vi "150pt Mov Avg.vi"(10 "Value in":dbl) -> (2 "Value out":dbl)   [LabVIEW 2014]
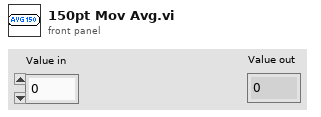
[diagram p1: front panel]
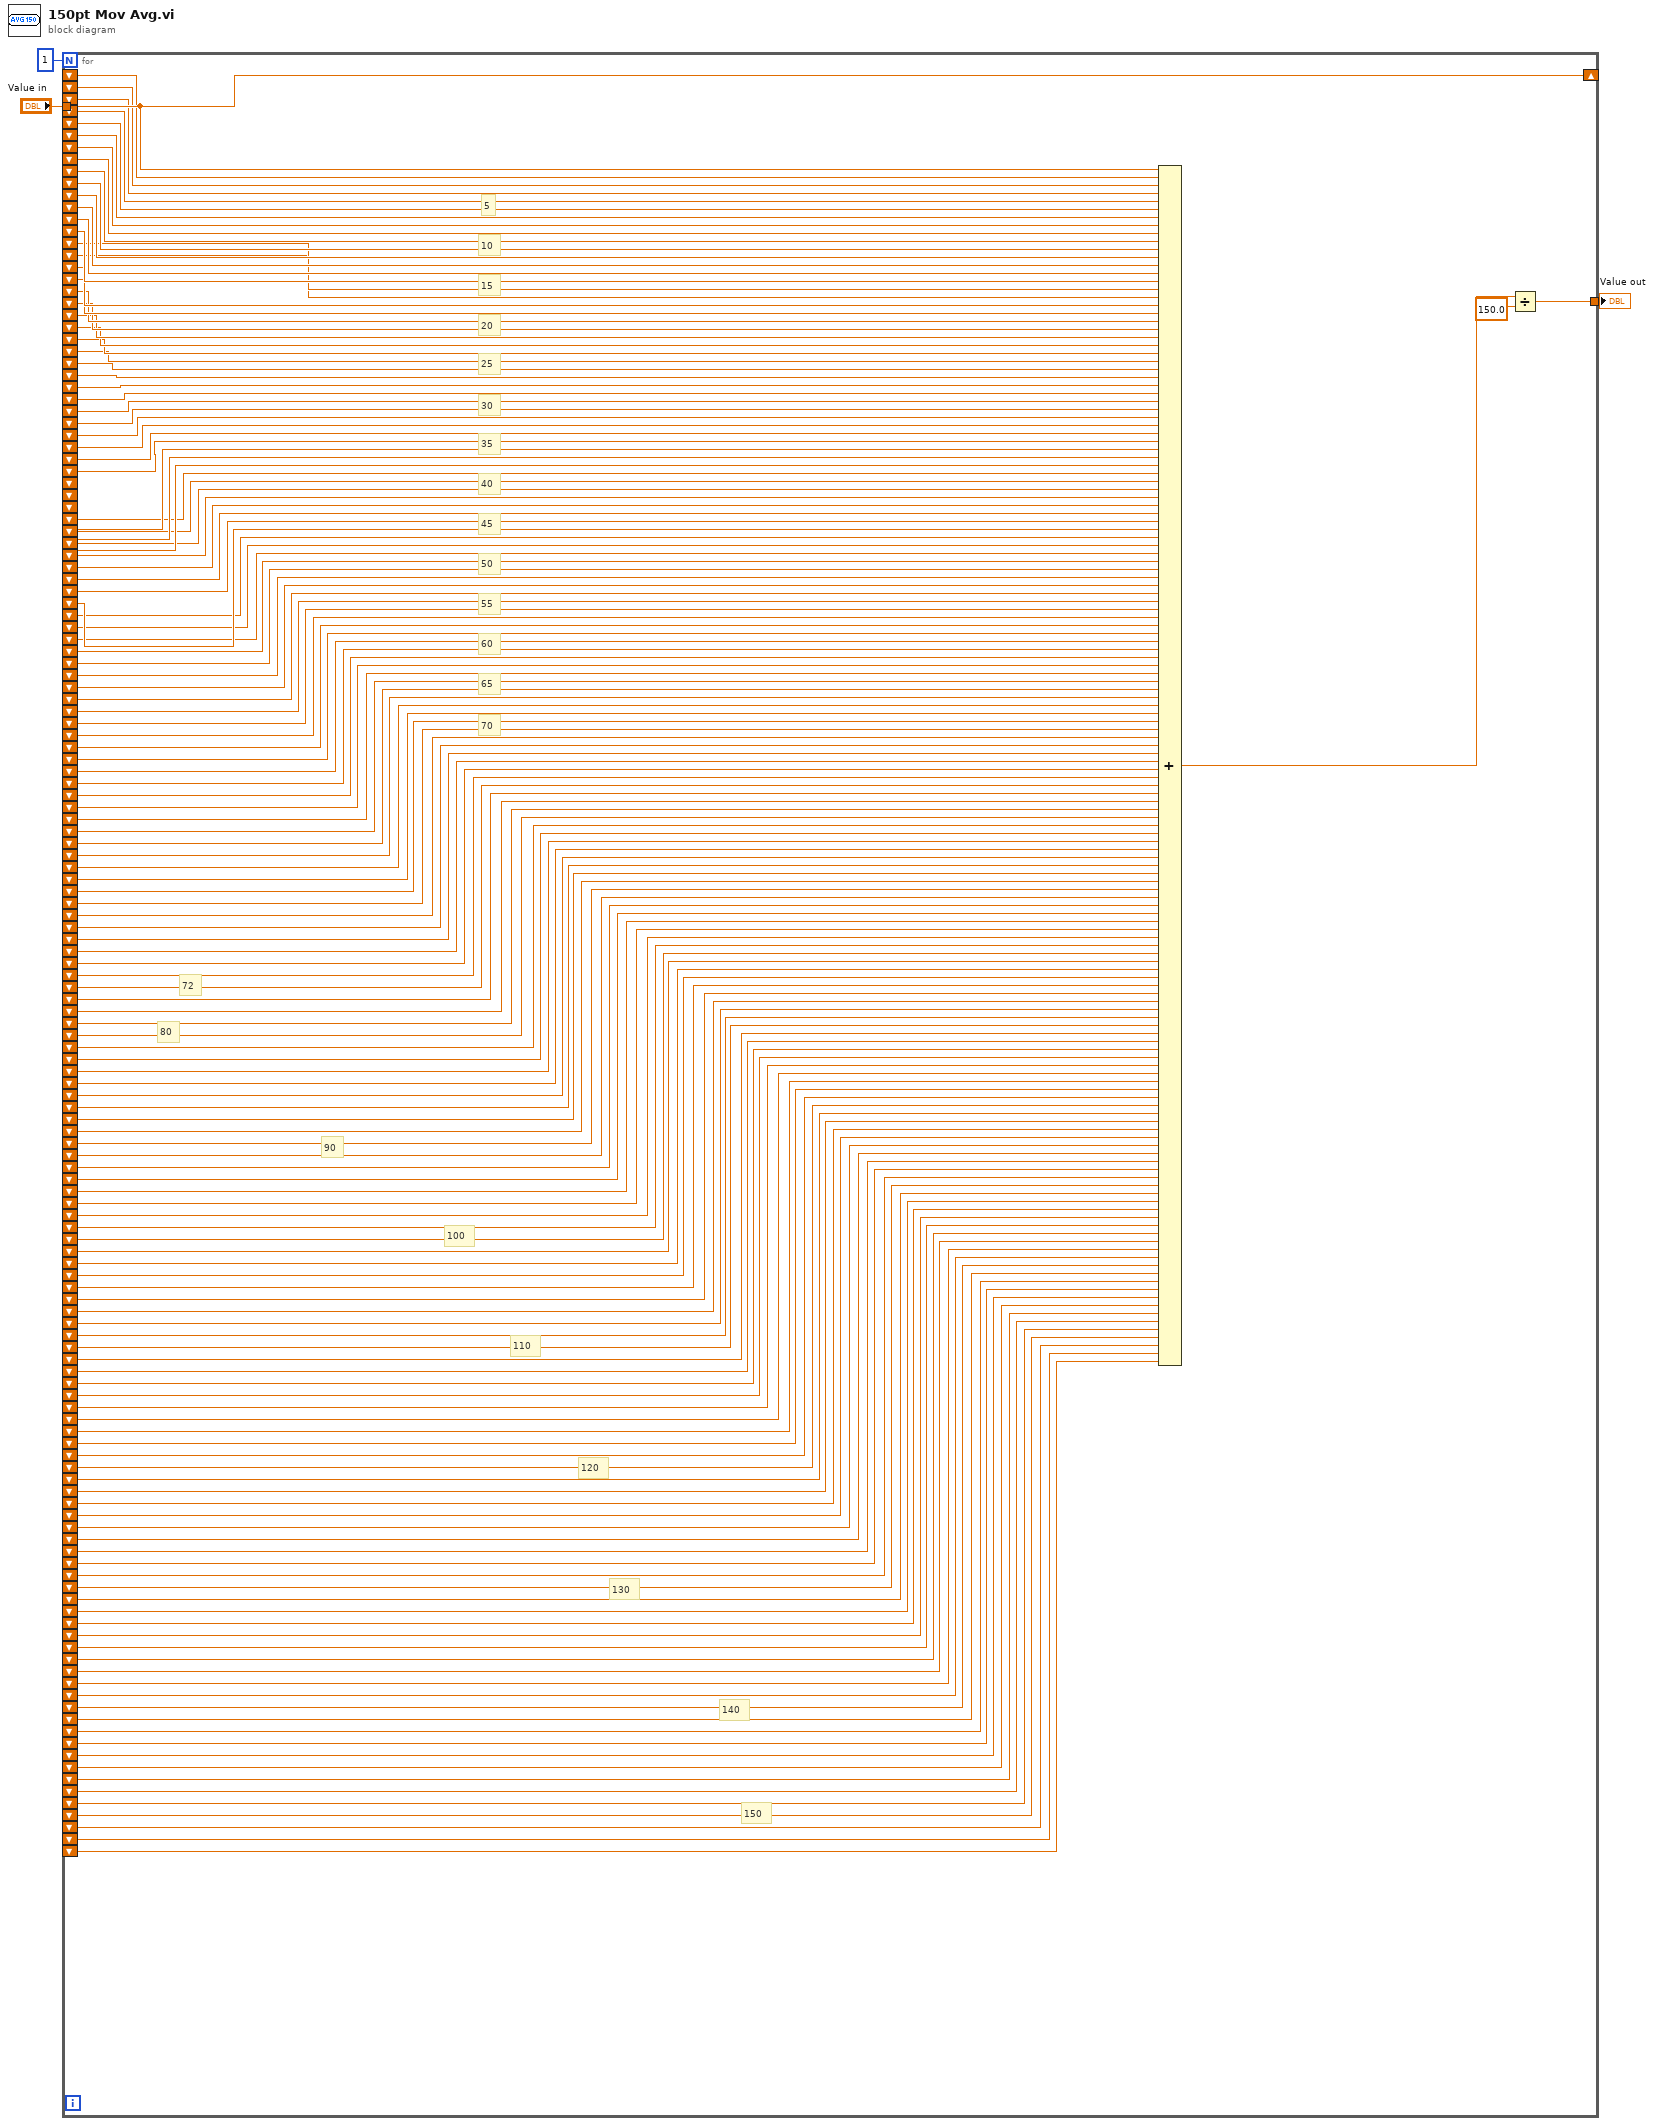
[diagram p0: block diagram]
diagram:
  n1 = for {
    N: 1 -> [_]
    tunnel: "Value in" -> [w156]
    shift-right: [w156] -> _
    shift-left: _ -> [w155]
    shift-left: _ -> [w154]
    shift-left: _ -> [w153]
    shift-left: _ -> [w152]
    tunnel: [w149] -> w1
    shift-left: _ -> [w148]
    shift-left: _ -> [w147]
    shift-left: _ -> [w146]
    shift-left: _ -> [w145]
    shift-left: _ -> [w144]
    shift-left: _ -> [w143]
    shift-left: _ -> [w142]
    shift-left: _ -> [w141]
    shift-left: _ -> [w140]
    shift-left: _ -> [w139]
    shift-left: _ -> [w138]
    shift-left: _ -> [w137]
    shift-left: _ -> [w136]
    shift-left: _ -> [w135]
    shift-left: _ -> [w134]
    shift-left: _ -> [w133]
    shift-left: _ -> [w132]
    shift-left: _ -> [w131]
    shift-left: _ -> [w130]
    shift-left: _ -> [w129]
    shift-left: _ -> [w128]
    shift-left: _ -> [w127]
    shift-left: _ -> [w126]
    shift-left: _ -> [w125]
    shift-left: _ -> [w124]
    shift-left: _ -> [w123]
    shift-left: _ -> [w122]
    shift-left: _ -> [w121]
    shift-left: _ -> [w120]
    shift-left: _ -> [w119]
    shift-left: _ -> [w118]
    shift-left: _ -> [w117]
    shift-left: _ -> [w116]
    shift-left: _ -> [w115]
    shift-left: _ -> [w113]
    shift-left: _ -> [w114]
    shift-left: _ -> [w112]
    shift-left: _ -> [w111]
    shift-left: _ -> [w110]
    shift-left: _ -> [w109]
    shift-left: _ -> [w108]
    shift-left: _ -> [w107]
    shift-left: _ -> [w106]
    shift-left: _ -> [w105]
    shift-left: _ -> [w104]
    shift-left: _ -> [w103]
    shift-left: _ -> [w102]
    shift-left: _ -> [w101]
    shift-left: _ -> [w100]
    shift-left: _ -> [w99]
    shift-left: _ -> [w98]
    shift-left: _ -> [w97]
    shift-left: _ -> [w96]
    shift-left: _ -> [w95]
    shift-left: _ -> [w94]
    shift-left: _ -> [w93]
    shift-left: _ -> [w92]
    shift-left: _ -> [w91]
    shift-left: _ -> [w90]
    shift-left: _ -> [w89]
    shift-left: _ -> [w88]
    shift-left: _ -> [w87]
    shift-left: _ -> [w86]
    shift-left: _ -> [w85]
    shift-left: _ -> [w84]
    shift-left: _ -> [w83]
    shift-left: _ -> [w82]
    shift-left: _ -> [w81]
    shift-left: _ -> [w80]
    shift-left: _ -> [w79]
    shift-left: _ -> [w78]
    shift-left: _ -> [w77]
    shift-left: _ -> [w76]
    shift-left: _ -> [w75]
    shift-left: _ -> [w74]
    shift-left: _ -> [w73]
    shift-left: _ -> [w72]
    shift-left: _ -> [w71]
    shift-left: _ -> [w70]
    shift-left: _ -> [w69]
    shift-left: _ -> [w68]
    shift-left: _ -> [w67]
    shift-left: _ -> [w66]
    shift-left: _ -> [w65]
    shift-left: _ -> [w64]
    shift-left: _ -> [w63]
    shift-left: _ -> [w62]
    shift-left: _ -> [w61]
    shift-left: _ -> [w60]
    shift-left: _ -> [w59]
    shift-left: _ -> [w58]
    shift-left: _ -> [w57]
    shift-left: _ -> [w56]
    shift-left: _ -> [w55]
    shift-left: _ -> [w54]
    shift-left: _ -> [w53]
    shift-left: _ -> [w52]
    shift-left: _ -> [w51]
    shift-left: _ -> [w50]
    shift-left: _ -> [w49]
    shift-left: _ -> [w48]
    shift-left: _ -> [w47]
    shift-left: _ -> [w46]
    shift-left: _ -> [w45]
    shift-left: _ -> [w44]
    shift-left: _ -> [w43]
    shift-left: _ -> [w42]
    shift-left: _ -> [w41]
    shift-left: _ -> [w40]
    shift-left: _ -> [w39]
    shift-left: _ -> [w38]
    shift-left: _ -> [w37]
    shift-left: _ -> [w36]
    shift-left: _ -> [w35]
    shift-left: _ -> [w34]
    shift-left: _ -> [w33]
    shift-left: _ -> [w32]
    shift-left: _ -> [w31]
    shift-left: _ -> [w30]
    shift-left: _ -> [w29]
    shift-left: _ -> [w28]
    shift-left: _ -> [w27]
    shift-left: _ -> [w26]
    shift-left: _ -> [w25]
    shift-left: _ -> [w24]
    shift-left: _ -> [w23]
    shift-left: _ -> [w22]
    shift-left: _ -> [w21]
    shift-left: _ -> [w20]
    shift-left: _ -> [w19]
    shift-left: _ -> [w18]
    shift-left: _ -> [w17]
    shift-left: _ -> [w16]
    shift-left: _ -> [w15]
    shift-left: _ -> [w14]
    shift-left: _ -> [w13]
    shift-left: _ -> [w12]
    shift-left: _ -> [w11]
    shift-left: _ -> [w10]
    shift-left: _ -> [w9]
    shift-left: _ -> [w8]
    shift-left: _ -> [w7]
    shift-left: _ -> [w6]
    shift-left: _ -> [w5]
    shift-left: _ -> [w4]
    # "150"
    # "140"
    # "130"
    # "120"
    # "110"
    # "100"
    # "90"
    # "80"
    # "72"
    # "70"
    # "65"
    # "55"
    # "45"
    # "35"
    # "30"
    # "25"
    # "20"
    # "15"
    # "10"
    # "5"
    # "60"
    # "50"
    # "40"
    n2 = Compound Arithmetic op=ADD(w156, w155, w154, w153, w152, w148, w147, w146, w145, w144, w143, w142, w141, w140, w139, w138, w137, w136, w135, w134, w133, w132, w131, w130, w129, w128, w127, w126, w125, w124, w123, w122, w121, w120, w119, w118, w117, w116, w115, w113, w114, w112, w111, w110, w109, w108, w107, w106, w105, w104, w103, w102, w101, w100, w99, w98, w97, w96, w95, w94, w93, w92, w91, w90, w89, w88, w87, w86, w85, w84, w83, w82, w81, w80, w79, w78, w77, w76, w75, w74, w73, w72, w71, w70, w69, w68, w67, w66, w65, w64, w63, w62, w61, w60, w59, w58, w57, w56, w55, w54, w53, w52, w51, w50, w49, w48, w47, w46, w45, w44, w43, w42, w41, w40, w39, w38, w37, w36, w35, w34, w33, w32, w31, w30, w29, w28, w27, w26, w25, w24, w23, w22, w21, w20, w19, w18, w17, w16, w15, w14, w13, w12, w11, w10, w9, w8, w7, w6, w5, w4) -> (w151:dbl)
    n3 = Divide(x=w151, y=150.0) -> (x/y=w149:dbl)
  }
  "Value out" <- w1
